vi "Help.Page.Get.vi"(11 "GUID":string) -> (2 "HTML File":string="PIDs.html")   [LabVIEW 2015, in "Diagnostics Addon System Explorer.lvlib"]
uses:
  Diagnostics Addon System Explorer.lvlib
  Shared/SubVIs/Constants.vi
  Shared/Diagnostics Addon Shared.lvlib
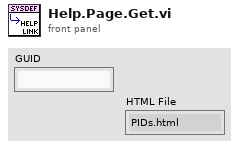
[diagram p1: front panel]
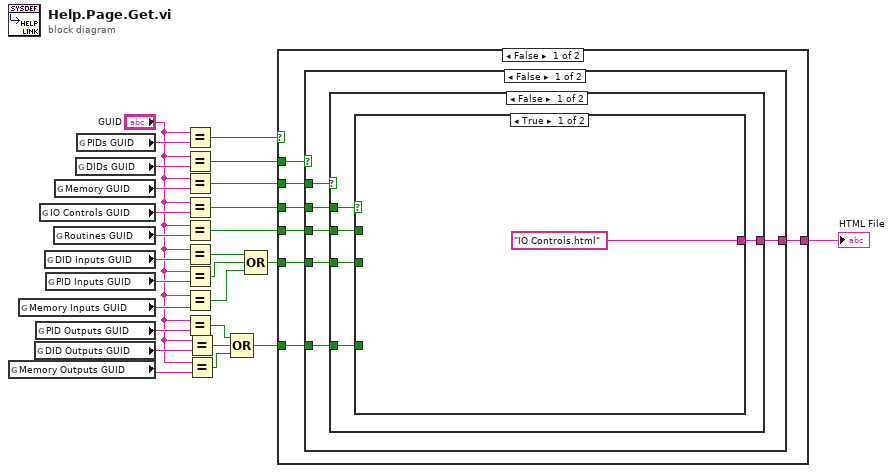
[diagram p0: block diagram]
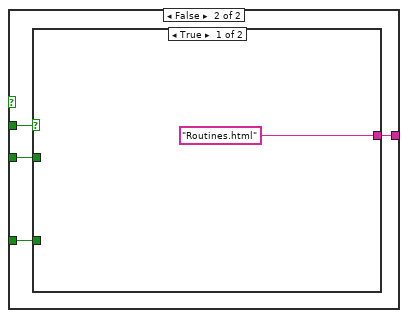
[diagram p2: hidden frame]
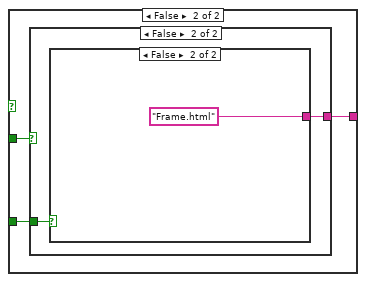
[diagram p3: hidden frame]
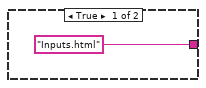
[diagram p4: hidden frame]
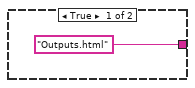
[diagram p5: hidden frame]
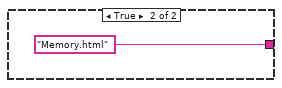
[diagram p6: hidden frame]
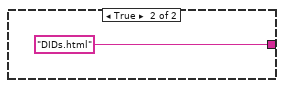
[diagram p7: hidden frame]
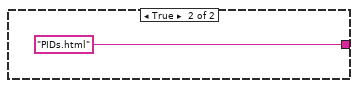
[diagram p8: hidden frame]
diagram:
  n1 = global read "Constants.vi" "Memory Outputs GUID"() -> (w4:string)
  n2 = global read "Constants.vi" "Memory Inputs GUID"() -> (w14:string)
  n3 = global read "Constants.vi" "DID Outputs GUID"() -> (w5:string)
  n4 = global read "Constants.vi" "PID Outputs GUID"() -> (w15:string)
  n5 = global read "Constants.vi" "IO Controls GUID"() -> (w22:string)
  n6 = global read "Constants.vi" "DID Inputs GUID"() -> (w13:string)
  n7 = global read "Constants.vi" "PID Inputs GUID"() -> (w12:string)
  n8 = global read "Constants.vi" "Routines GUID"() -> (w21:string)
  n9 = global read "Constants.vi" "Memory GUID"() -> (w26:string)
  n10 = global read "Constants.vi" "DIDs GUID"() -> (w25:string)
  n11 = global read "Constants.vi" "PIDs GUID"() -> (w24:string)
  n12 = Equal?(x="GUID", y=w24) -> (x = y?=w20:bool)
  n13 = Equal?(x="GUID", y=w25) -> (x = y?=w19:bool)
  n14 = Equal?(x="GUID", y=w26) -> (x = y?=w18:bool)
  n15 = Equal?(x="GUID", y=w22) -> (x = y?=w17:bool)
  n16 = Equal?(x="GUID", y=w21) -> (x = y?=w16:bool)
  n17 = Equal?(x="GUID", y=w13) -> (x = y?=w11:bool)
  n18 = Equal?(x="GUID", y=w12) -> (x = y?=w10:bool)
  n19 = Equal?(x="GUID", y=w14) -> (x = y?=w9:bool)
  n20 = Equal?(x="GUID", y=w15) -> (x = y?=w2:bool)
  n21 = Equal?(x="GUID", y=w5) -> (x = y?=w6:bool)
  n22 = Equal?(x="GUID", y=w4) -> (x = y?=w7:bool)
  n23 = Compound Arithmetic op=OR(w2, w6, w7) -> (w1:bool)
  n24 = Compound Arithmetic op=OR(w11, w10, w9) -> (w8:bool)
  n25 = case shown="False" w20 {
    tunnel: [w33 "PIDs.html" ("HTML File")] -> w23
    tunnel: w19 -> [w32 _]
    tunnel: w18 -> [w31 _]
    tunnel: w17 -> [w30 _]
    tunnel: w16 -> [w29 _]
    tunnel: w8 -> [w28 _]
    tunnel: w1 -> [w27 _]
    frame False {
      n26 = case shown="False" w32 {
        tunnel: [w39 "DIDs.html" ("HTML File")] -> w33
        tunnel: w31 -> [w38 _]
        tunnel: w30 -> [w37 _]
        tunnel: w29 -> [w36 _]
        tunnel: w28 -> [w35 _]
        tunnel: w27 -> [w34 _]
        frame False {
          n27 = case shown="False" w38 {
            tunnel: [w44 "Memory.html" ("HTML File")] -> w39
            tunnel: w37 -> [w43 _]
            tunnel: w36 -> [w42 _]
            tunnel: w35 -> [w41 _]
            tunnel: w34 -> [w40 _]
            frame False {
              n28 = case shown="True" w43 {
                tunnel: ["IO Controls.html" ("HTML File") w49] -> w44
                tunnel: w42 -> [_ w48]
                tunnel: w41 -> [_ w47]
                tunnel: w40 -> [_ w46]
                frame True {
                }
                frame False {
                  n29 = case shown="True" w48 {
                    tunnel: ["Routines.html" ("HTML File") w53] -> w49
                    tunnel: w47 -> [_ w52]
                    tunnel: w46 -> [_ w51]
                    frame True {
                    }
                    frame False {
                      n30 = case shown="False" w52 {
                        tunnel: ["Inputs.html" ("HTML File") w56] -> w53
                        tunnel: w51 -> [_ w55]
                        frame True {
                        }
                        frame False {
                          n31 = case shown="False" w55 {
                            tunnel: ["Outputs.html" ("HTML File") "Frame.html" ("HTML File")] -> w56
                            frame True {
                            }
                            frame False {
                            }
                          }
                        }
                      }
                    }
                  }
                }
              }
            }
            frame True {
            }
          }
        }
        frame True {
        }
      }
    }
    frame True {
    }
  }
  "HTML File" <- w23
